vi "Coherent comms L1.vi"(7 "Coherent laser commands L1":T4(ring), 8 "error in (no error)":errorcluster, 9 "Data":T2, 10 "Commands & Queries":T5, 11 "Visa resource":T3) -> (0 "error out":errorcluster, 1 "Data Type":T1, 3 "Response":string)   [LabVIEW 2020]
uses:
  Type defs/Commands List.ctl
  Serial Comms/Visa resource.ctl
  Type defs/data type.ctl
  Serial Comms/Serial - Settings.ctl
panel:
  out "Output":string
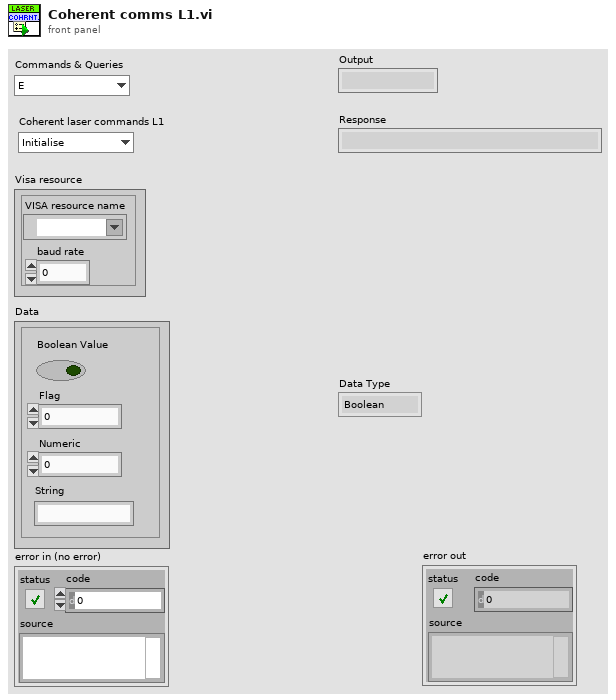
[diagram p1: front panel]
types:
  T1 = typedef "data type.ctl" = enum16{"Boolean", "Flag", "Numeric", "String", "Array"}
  T2 = cluster{"Boolean Value":bool, "Flag":i32, "Numeric":dbl, "String":string}
  T3 = typedef "Visa resource.ctl" = cluster{"VISA resource name":refnum<visa-resource-name>, "baud rate":u32}
  T4 = enum16{"Initialise", "Get Command", "Set Command", "Close"}
  T5 = typedef "Commands List.ctl" = enum16{"E", "B", "FL", "HM", "L", "LBOH", "LBOOPT", "LFP", "PROMPT", "SM", "S", "VW", "VWS", "HB", "HBR", "REQ", "ALIGN", "K", "F", "FH", "UF", "PHLDC", "PZTMC", "PZTXC", "PZTYC", "PHLDP", "PZTMP", "PZTXP", "PZTYP", "PTRK", "MDLK", "PP", "TS", "STPRPOS", "C", "D1C", "D2C", "BT", "D1T", "D2T", "VT", "LBOT", "ET", "D1ST", "D2ST", "VST", "LBOST", "EST", "D1TD", "D2TD", "VD", "LBOD", "ED", "D1HST", "D2HST", "LRS", "D1SS", "D2SS", "VSS", "LBOSS", "ESS", "D1H", "D2H", "HH", "D1V", "D2V", "SV", "MB", "PI", "BV", "AMDLK", "PZTS", "TMAX", "TMIN", "ALIGNP", "ALIGNW", "PZTXCM", "PZTXCP", "PZTXPM", "PZTXPP", "PZTYCM", "PZTYCP", "PZTYPM", "PZTYPP", "RH", "SN", "ST", "GDDCURVE", "GDD", "GDDCURVEN", "SETCURVEN", "SETCURVEPT", "SAVECURVE", "DELCURVE", "CURVEN", "CURVEPT", "CURVE", "COMP", "HMCOMP", "GDDMAX", "GDDMIN"}
  T6 = enum16{"Initialise", "Read Handle", "Command & Query", "Close"}
  T7 = typedef "Serial - Settings.ctl" = cluster{"VISA resource name ":refnum<visa-resource-name>, "baud rate":u32, "data bits":u16, "parity":enum16{"None", "Odd", "Even", "Mark", "Space"}, "stop bits":u16, "flow control":u16}
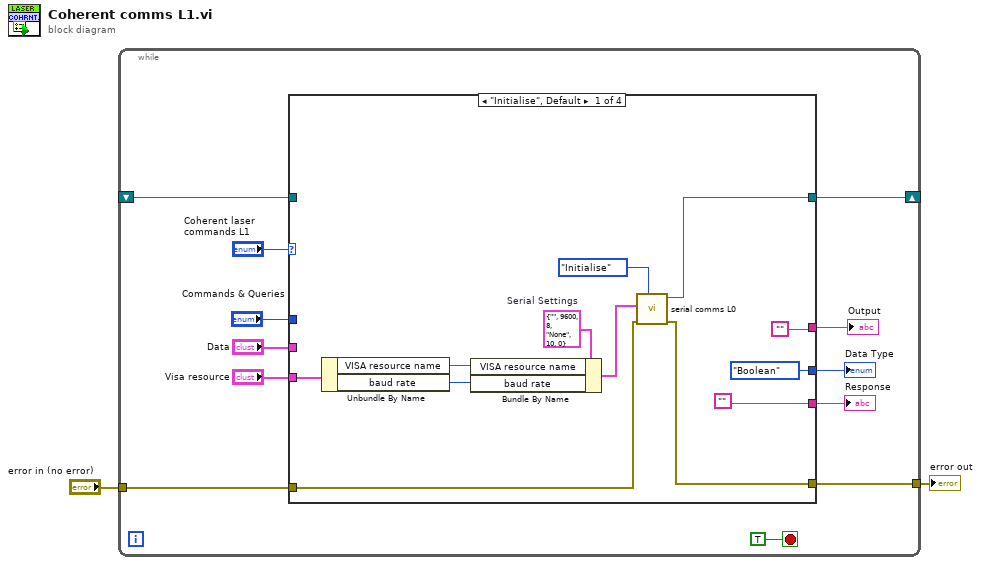
[diagram p0: block diagram]
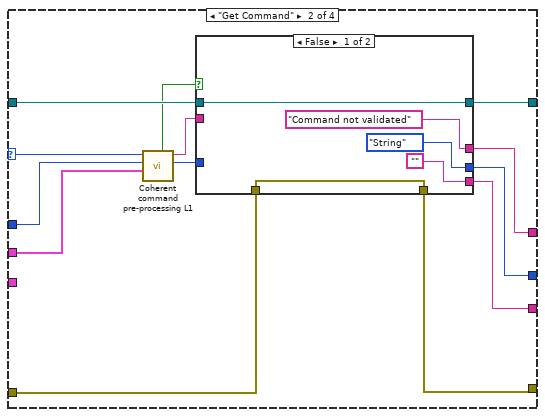
[diagram p2: hidden frame]
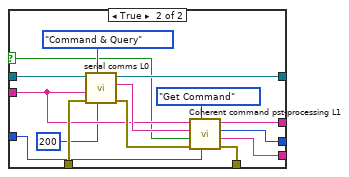
[diagram p3: hidden frame]
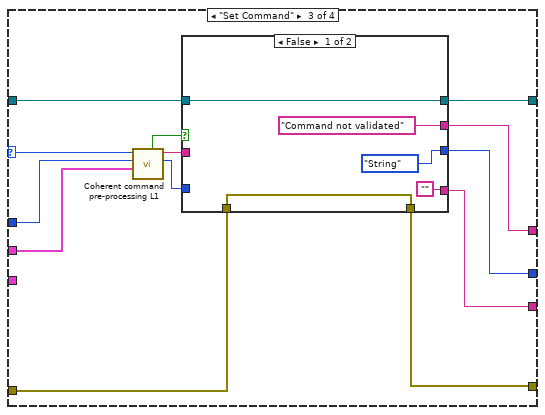
[diagram p4: hidden frame]
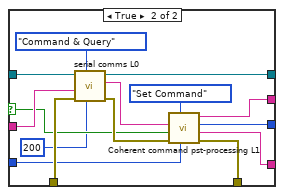
[diagram p5: hidden frame]
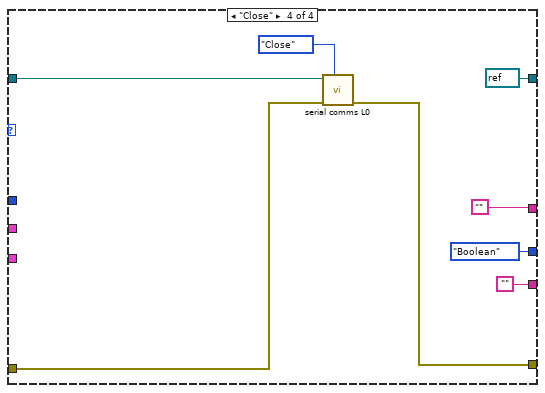
[diagram p6: hidden frame]
diagram:
  n1 = while {
    tunnel: "error in (no error)" -> [w13]
    tunnel: [w12] -> w1
    shift-right: [w8] -> _
    shift-left: _ -> [w6]
    stop <- TRUE stop-if-true
    n2 = case shown="\"Initialise\", Default" "Coherent laser commands L1" {
      selector: "Coherent laser commands L1" -> [_ w39 w72 _]
      tunnel: w13 -> [w24 w33 w66 w98]
      tunnel: [w23 w28 w65 w97] -> w12
      tunnel: "Visa resource" -> [w22 _ _ _]
      tunnel: "Data" -> [_ w37 w70 _]
      tunnel: [w19 w35 w68 refnum<visa-resource-name> refnum ("VISA resource name out")] -> w8
      tunnel: "Commands & Queries" -> [_ w38 w71 _]
      tunnel: w6 -> [_ w36 w69 w99]
      tunnel: ["" w32 w64 ""] -> w5
      tunnel: [data_type."Boolean" ("Data Type") w30 w61 data_type."Boolean" ("Data Type")] -> w4
      tunnel: ["" w27 w60 ""] -> w3
      frame "Initialise", Default {
        w26 = T7 {"VISA resource name "="", "baud rate"=9600, "data bits"=8, "parity"=enum."None", "stop bits"=10, "flow control"=0}  # Serial Settings
        n3 = Unbundle By Name(w22) -> ("VISA resource name"=w21:refnum<visa-resource-name>, "baud rate"=w20:u32)
        n4 = Bundle By Name(cluster=w26, "VISA resource name"=w21, "baud rate"=w20) -> (w25:T7)
        n5 = call "serial comms L0.vi"("Comms Control"=T6."Initialise", "error IN"=w24, "Serial Settings"=w25) -> ("Error OUT"=w23:errorcluster, "VISA resource name out"=w19:refnum<visa-resource-name>)  [unwired: 3 in, 4 out]
      }
      frame "Get Command" {
        n6 = call "Coherent command pre-processing L1.vi"("Data"=w37, "Commands & Queries"=w38, "Coherent laser commands L1"=w39) -> ("Data Type"=w29:T1, "Command/Query string"=w34:string, "Command validated ?"=w31:bool)  [unwired: 6 in]
        n7 = case shown="False" w31 {
          selector: w31 -> [_ w49]
          tunnel: w36 -> [w44 w59]
          tunnel: [w44 w58] -> w35
          tunnel: w34 -> [_ w51]
          tunnel: w33 -> [w42 w56]
          tunnel: ["" w53] -> w32
          tunnel: [data_type."String" ("Data Type") w52] -> w30
          tunnel: w29 -> [_ w48]
          tunnel: [w42 w47] -> w28
          tunnel: ["Command not validated" w45] -> w27
          frame False {
          }
          frame True {
            n8 = call "serial comms L0.vi"("delay before read (ms)"=u32 200, "Comms Control"=T6."Command & Query", "error IN"=w56, "Command String"=w51, "VISA resource name"=w59) -> ("Error OUT"=w55:errorcluster, "Response"=w54:string, "VISA resource name out"=w58:refnum<visa-resource-name>)  [unwired: 1 in, 3 out]
            n9 = call "Coherent command pst-processing L1.vi"("Data Type"=w48, "Coherent laser commands L1"=T4."Get Command", "error in (no error)"=w55, "Command Validated"=w49, "Response String"=w54, "Command String"=w51) -> ("error out"=w47:errorcluster, "Response String"=w53:string, "Data Type"=w52:T1, "trimmed string"=w45:string)  [unwired: 2 in]
          }
        }
      }
      frame "Set Command" {
        n10 = call "Coherent command pre-processing L1.vi"("Data"=w70, "Commands & Queries"=w71, "Coherent laser commands L1"=w72) -> ("Data Type"=w62:T1, "Command/Query string"=w67:string, "Command validated ?"=w63:bool)  [unwired: 6 in]
        n11 = case shown="False" w63 {
          selector: w63 -> [_ w84]
          tunnel: w69 -> [w77 w92]
          tunnel: [w77 w91] -> w68
          tunnel: w67 -> [_ w89]
          tunnel: w66 -> [w75 w88]
          tunnel: [w75 w81] -> w65
          tunnel: ["" w82] -> w64
          tunnel: w62 -> [_ w83]
          tunnel: [data_type."String" ("Data Type") w80] -> w61
          tunnel: ["Command not validated" ("String") w78] -> w60
          frame False {
          }
          frame True {
            n12 = call "serial comms L0.vi"("delay before read (ms)"=u32 200, "Comms Control"=T6."Command & Query", "error IN"=w88, "Command String"=w89, "VISA resource name"=w92) -> ("Error OUT"=w85:errorcluster, "Response"=w86:string, "VISA resource name out"=w91:refnum<visa-resource-name>)  [unwired: 1 in, 3 out]
            n13 = call "Coherent command pst-processing L1.vi"("Data Type"=w83, "Coherent laser commands L1"=T4."Set Command", "error in (no error)"=w85, "Command Validated"=w84, "Response String"=w86) -> ("error out"=w81:errorcluster, "Response String"=w82:string, "Data Type"=w80:T1, "trimmed string"=w78:string)  [unwired: 3 in]
          }
        }
      }
      frame "Close" {
        n14 = call "serial comms L0.vi"("Comms Control"=T6."Close", "error IN"=w98, "VISA resource name"=w99) -> ("Error OUT"=w97:errorcluster)  [unwired: 3 in, 5 out]
      }
    }
    "Response" <- w5
    "Data Type" <- w4
    "Output" <- w3
  }
  "error out" <- w1
